vi "Butterfly_PullDown RC2_wCap_ERMod.vi"(0 "Semiconductor Module Context":T2, 1 "RFPins":string[](array[string]), 2 "current level":dbl=0.01 format="%_6p", 3 "R Thresholds":dbl[](array[numeric]), 5 "error in (no error)":errorcluster, 6 "PD_Pin":string="SMU_PD", 7 "Start_v":dbl=10.0 format="%#_13g", 9 "Stop_v":dbl=41.0 format="%#_13g", 10 "VNAs Measurement Parameters":T1, 11 "Step_v":dbl=1.0) -> (14 "Semiconductor Module Context Out":T2, 19 "error out":errorcluster)   [LabVIEW 2013]
uses:
  <vilib>/NI_TestStand_SemiconductorModule/NI_TestStand_Semiconductor_Module.lvlibp/PinMap/General/SemiconductorModuleContext.ctl
  VNA/VNAs Measurement Parameters.ctl
  <instrlib>/niDCPower/nidcpower.llb/niDCPower Wait For Event - Event.ctl
  <vilib>/NI_TestStand_SemiconductorModule/NI_TestStand_Semiconductor_Module.lvlibp/PinMap/DC Power/PinToNIDCPowerSession.vi
  <vilib>/NI_TestStand_SemiconductorModule/NI_TestStand_Semiconductor_Module.lvlibp/PinMap/DC Power/PinsToNIDCPowerSessions.vi
  <vilib>/NI_TestStand_SemiconductorModule/NI_TestStand_Semiconductor_Module.lvlibp/PinMap/General/Publish/PublishDataDoubleFunctionalTest.vi
  <vilib>/NI_TestStand_SemiconductorModule/NI_TestStand_Semiconductor_Module.lvlibp
panel:
  out "Multisite Cap Data":dbl[][](array[numeric])
  out "Full R Array":dbl[][][](array[numeric])
  out "step":i32
  out "Instrument Session":refnum<k15>
  out "sites and pins loop iter":i32
  out "Channel List":string
  out "BF values":dbl[](array[numeric])
  out "BF Names":string[](array[string])
  out "R Array":dbl[](array[numeric])
  out "BFSamples":i32
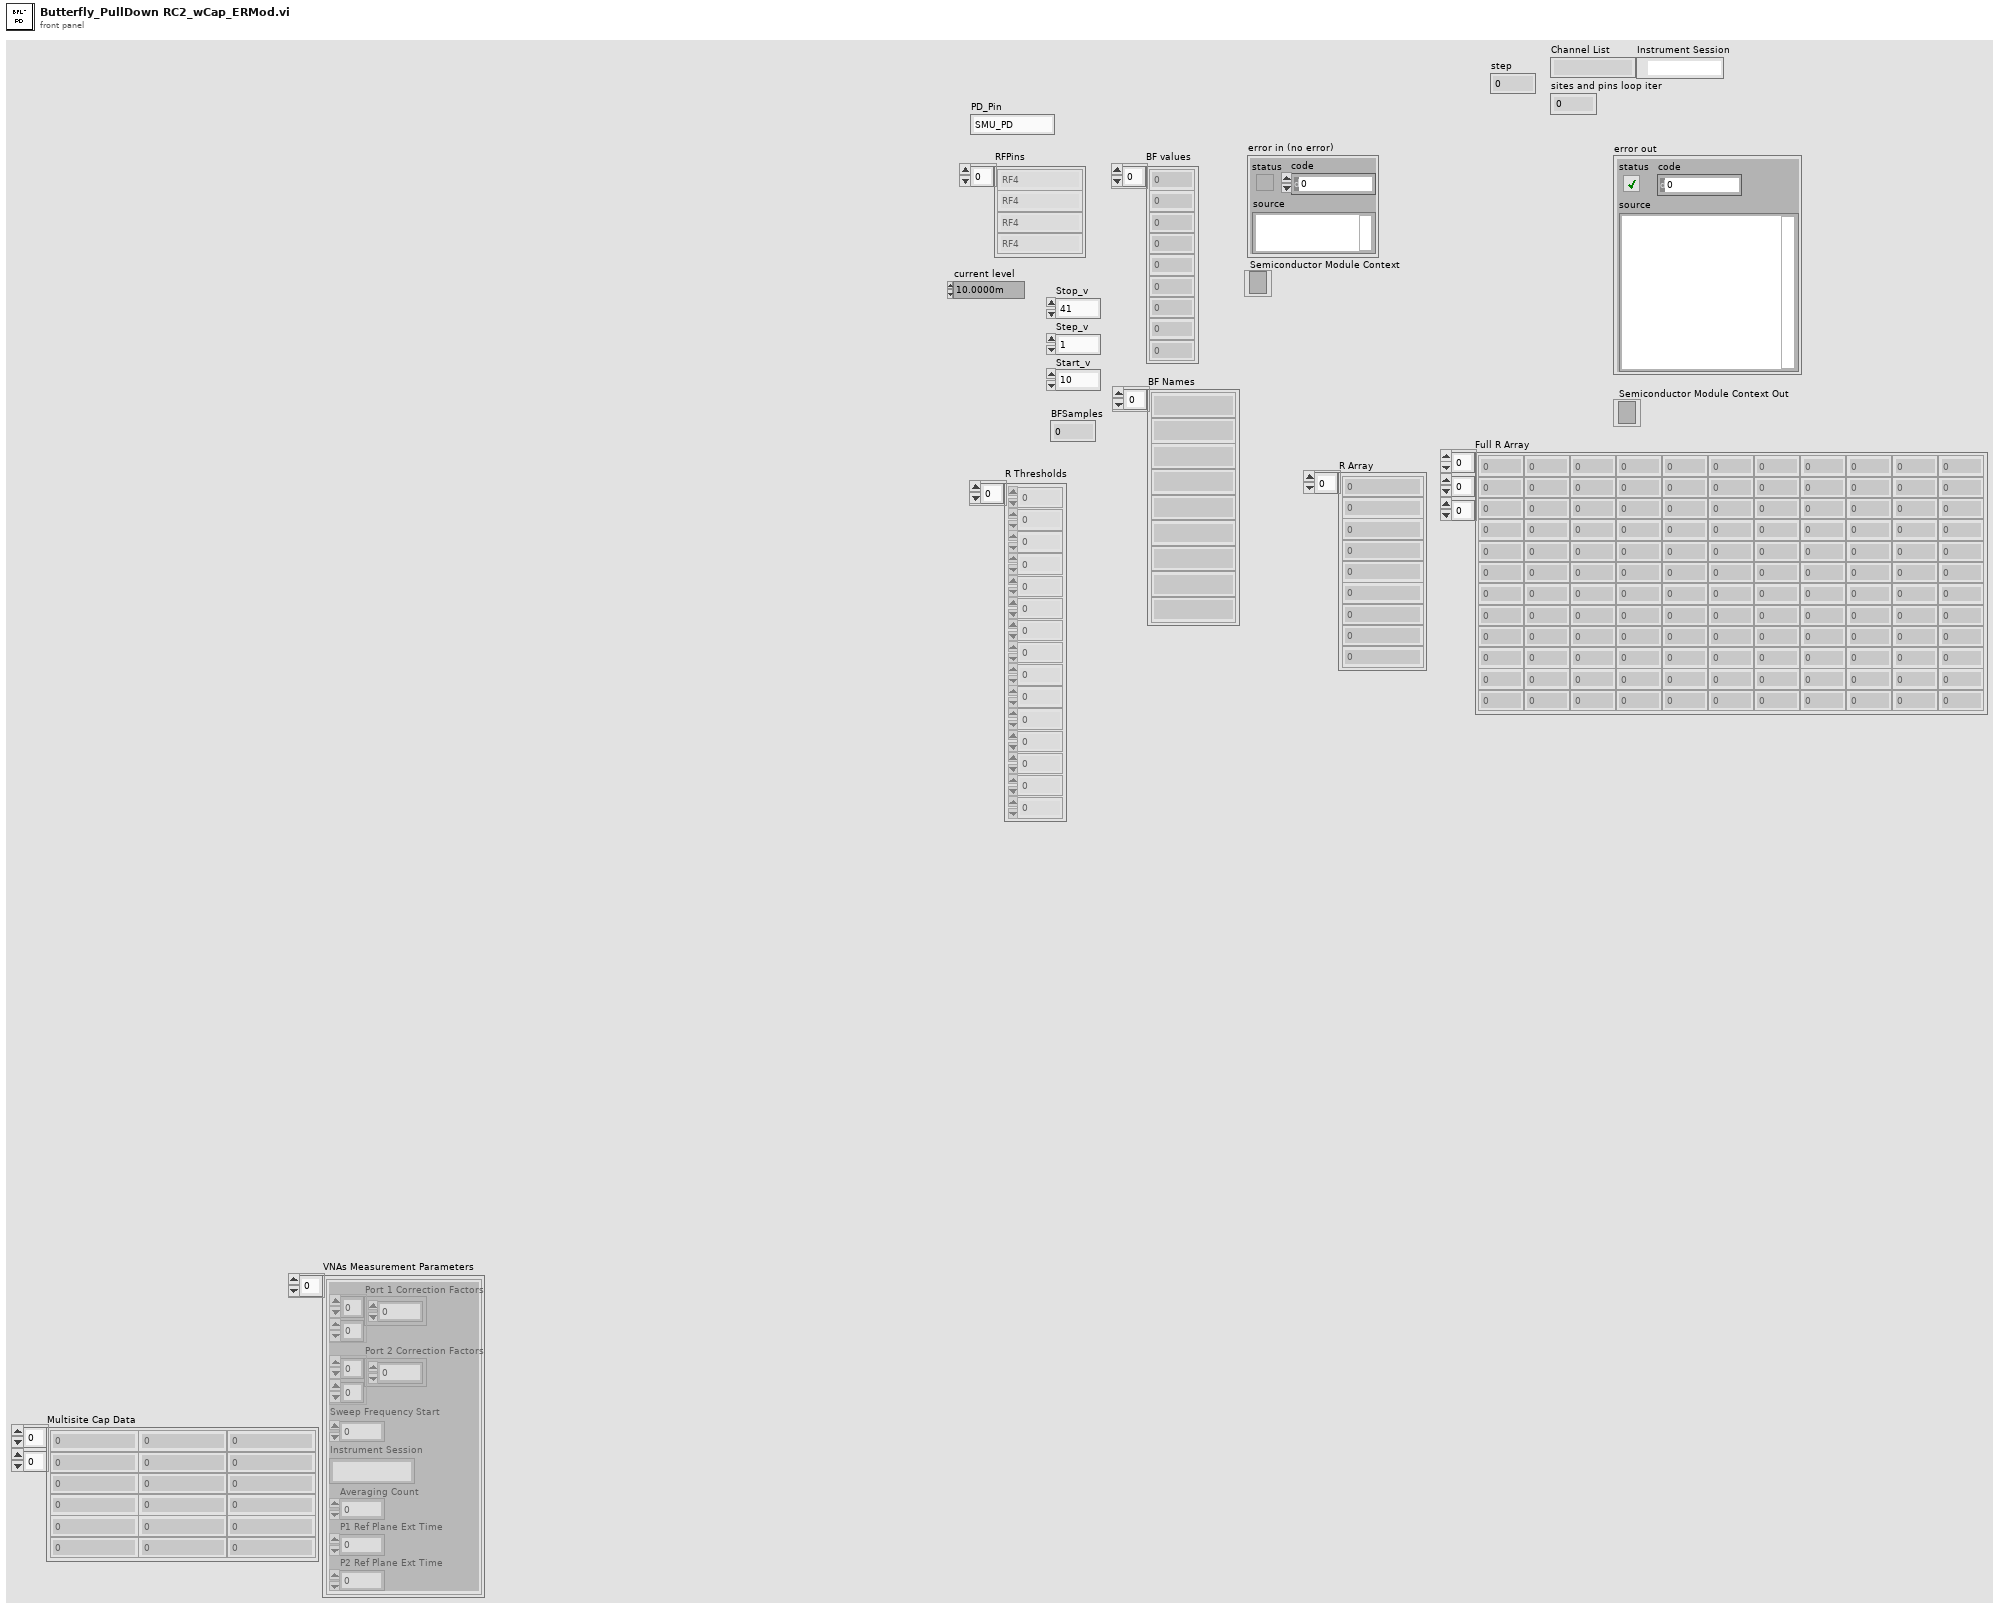
[diagram p1: front panel]
types:
  T1 = typedef "VNAs Measurement Parameters.ctl" = cluster{"Port 1 Correction Factors":cdb[][], "Port 2 Correction Factors":cdb[][], "Sweep Frequency Start":dbl, "Instrument Session":string, "Averaging Count":i32, "P1 Ref Plane Ext Time":dbl, "P2 Ref Plane Ext Time":dbl}[]
  T2 = typedef "NI_TestStand_Semiconductor_Module.lvlibp/SemiconductorModuleContext.ctl" = refnum<k7>
  T3 = typedef "niDCPower Wait For Event - Event.ctl" = i32
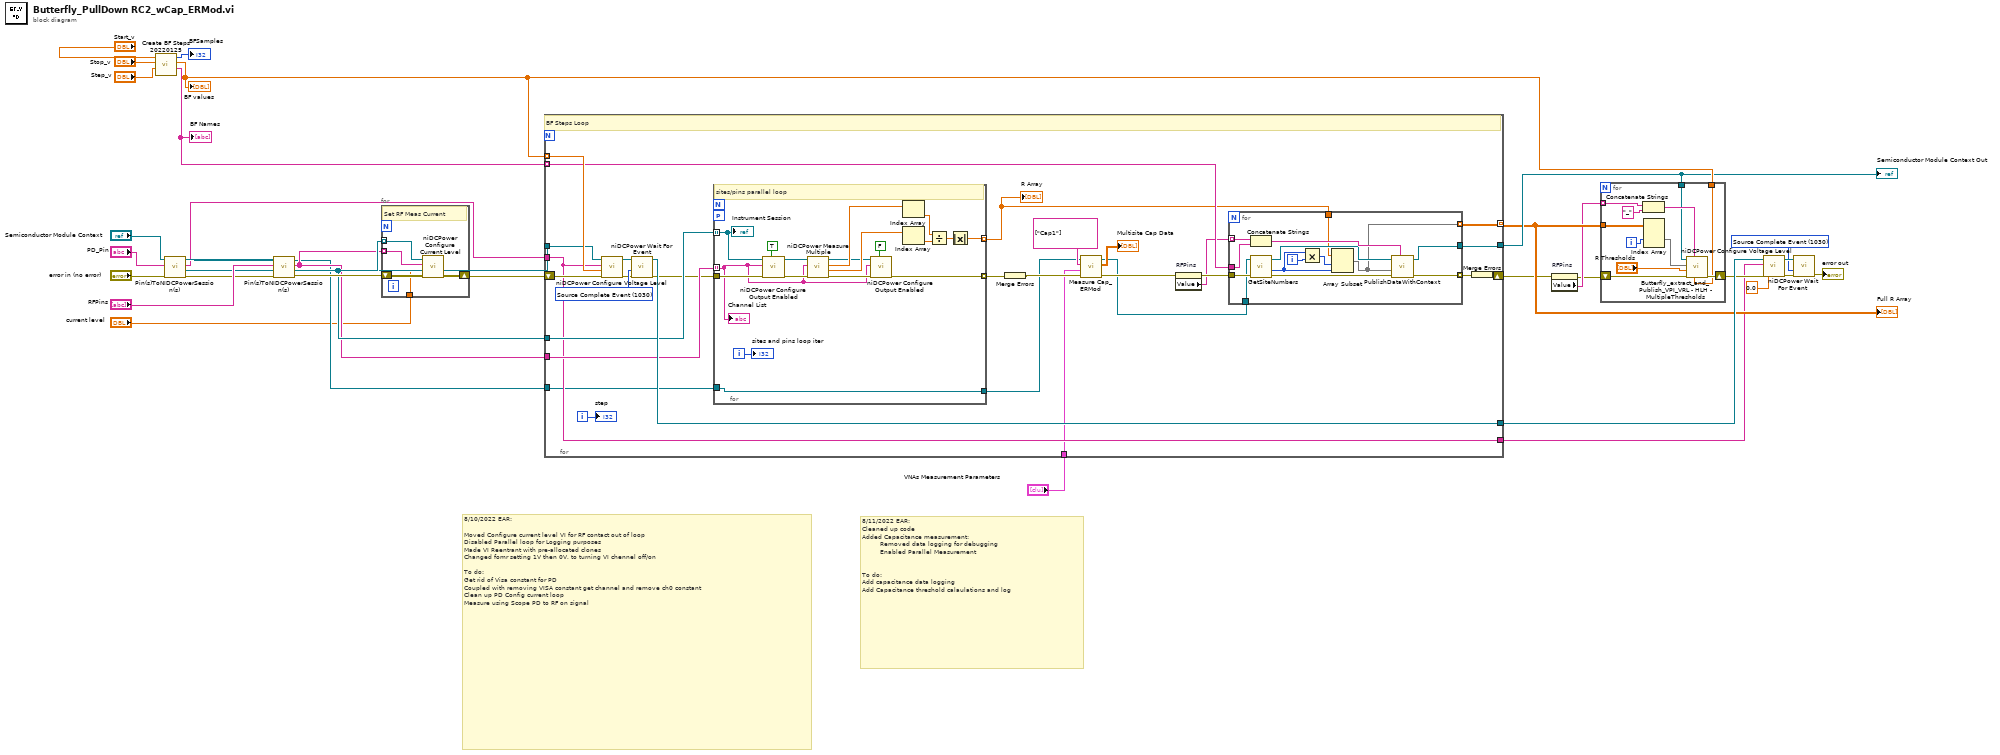
[diagram p0: block diagram]
diagram:
  w25 = T3 1030 items=["Source Complete Event"=1030, "Measure Complete Event"=1031, "Sequence Iteration Complete Event"=1032, "Sequence Engine Done Event"=1033, "Pulse Complete Event"=1051, "Ready For Pulse Trigger Event"=1052] ("event")
  # "8/11/2022 EAR:\nCleaned up code\nAdded Capacitance measurement:\n         Removed data logging for debugging\n         Enabled Parallel Measurement\n\n\nTo do:\nAdd capacitance data logging\nAdd Capacitance threshold calaulations and log"
  # "8/10/2022 EAR:\n\nMoved Configure current level VI for RF contact out of loop\nDisabled Parallel loop for Logging purposes\nMade VI Reentrant with pre-allocated clones\nChanged fomr setting 1V then 0V, to turning VI chennel off/on\n\nTo do:\nGet rid of Visa constant for PD\nCoupled with removing VISA constant get channel and remove ch0 constant\nClean up PD Config current loop\nMeasure using Scope PD to RF on signal"
  n1 = call "Create BF Steps 20220125.vi"("Step_v"="Step_v", "Stop_v"="Stop_v", "Start_v"="Start_v") -> ("BF Names"=w24:string[], "BF values"=w23:dbl[], "BFSamples"=→"BFSamples":i32)  [unwired: 6 in]
  "BF Names" <- w24
  "BF values" <- w23
  n2 = call-poly <vilib>:"Pin(s)ToNIDCPowerSession(s).vi"("error in (no error)"="error in (no error)", "Pin"="PD_Pin", "Semiconductor Module Context"="Semiconductor Module Context") -> ("error out"=w11:errorcluster, "Instrument Session"=w8:refnum<k15>, "Channel List"=w7:string, "Semiconductor Module Context Out"=w12:T2)  [unwired: 4 in, 1 out]
  n3 = call-poly <vilib>:"Pin(s)ToNIDCPowerSession(s).vi"("error in (no error)"=w11, "Pins"="RFPins", "Semiconductor Module Context"=w12) -> ("error out"=w20:errorcluster, "Instrument Sessions"=w18:refnum<k15>[], "Channel Lists"=w17:string[], "Semiconductor Module Context Out"=w15:T2)  [unwired: 4 in, 1 out]
  n4 = for {
    shift-right: [w38] -> w19
    shift-left: w20 -> [w39]
    tunnel: w18 -> [w37] mode=indexing
    tunnel: w17 -> [w36] mode=indexing
    tunnel: "current level" -> [w35]
    # "Set RF Meas Current"
    n5 = call <instrlib>:"niDCPower Configure Current Level.vi"("error in (no error)"=w39, "current level"=w35, "channel name"=w36, "instrument handle"=w37) -> ("error out"=w38:errorcluster)  [unwired: 6 in, 1 out]
  }
  n6 = for {
    shift-right: [w57] -> w4
    shift-left: w19 -> [w65]
    tunnel: w23 -> [w64] mode=indexing
    tunnel: w8 -> [w63]
    tunnel: [w62] -> w29
    tunnel: w24 -> [w59] mode=indexing
    tunnel: [w58] -> w21
    tunnel: w18 -> [w56]
    tunnel: w17 -> [w55]
    tunnel: w15 -> [w47]
    tunnel: [w52] -> w14 mode=indexing
    tunnel: w7 -> [w48]
    tunnel: [w48] -> w2
    tunnel: "VNAs Measurement Parameters" -> [w40]
    i -> [w61]
    w67 = T3 1030 items=["Source Complete Event"=1030, "Measure Complete Event"=1031, "Sequence Iteration Complete Event"=1032, "Sequence Engine Done Event"=1033, "Pulse Complete Event"=1051, "Ready For Pulse Trigger Event"=1052] ("event")
    # "BF Steps Loop"
    n7 = call <instrlib>:"niDCPower Configure Voltage Level.vi"("error in (no error)"=w65, "voltage level"=w64, "channel name"=w48, "instrument handle"=w63) -> ("error out"=w66:errorcluster, "instrument handle out"=w68:refnum<k15>)  [unwired: 6 in]
    n8 = call <instrlib>:"niDCPower Wait For Event.vi"("error in (no error)"=w66, "event"=w67, "instrument handle"=w68) -> ("error out"=w54:errorcluster, "instrument handle out"=w62:refnum<k15>)  [unwired: 7 in]
    n9 = for {
      workers-P: _ -> [_]
      tunnel: w56 -> [w90] mode=indexing
      tunnel: w55 -> [w86] mode=indexing
      tunnel: [w85] -> w53 mode=indexing
      tunnel: w54 -> [w94]
      tunnel: [w84] -> w51 mode=indexing
      tunnel: w47 -> [w83]
      tunnel: [w83] -> w42
      i -> [w100]
      # "sites/pins parallel loop"
      n10 = call <instrlib>:"niDCPower Configure Output Enabled.vi"("error in (no error)"=w94, "output enabled"=TRUE, "channel name"=w86, "instrument handle"=w90) -> ("error out"=w92:errorcluster, "instrument handle out"=w91:refnum<k15>)  [unwired: 6 in]
      n11 = call <instrlib>:"niDCPower Measure Multiple.vi"("error in (no error)"=w92, "channel name"=w86, "instrument handle"=w91) -> ("error out"=w89:errorcluster, "current measurements"=w99:dbl[], "voltage measurements"=w98:dbl[], "instrument handle out"=w87:refnum<k15>)  [unwired: 5 in]
      n12 = call <instrlib>:"niDCPower Configure Output Enabled.vi"("error in (no error)"=w89, "output enabled"=FALSE, "channel name"=w86, "instrument handle"=w87) -> ("error out"=w84:errorcluster)  [unwired: 6 in, 1 out]
      n13 = Index Array(array=w98) -> (element=w96:dbl)  [unwired: 1 in]
      n14 = Index Array(array=w99) -> (element=w97:dbl)  [unwired: 1 in]
      n15 = Divide(x=w96, y=w97) -> (x/y=w95:dbl)
      n16 = Absolute Value(x=w95) -> (abs(x)=w85:dbl)
      "Channel List" <- w86
      "sites and pins loop iter" <- w100
      "Instrument Session" <- w90
    }
    "R Array" <- w53
    n17 = Merge Errors(w51) -> (w44:errorcluster)
    n18 = call "Measure Cap_ERMod.vi"("error in (no error)"=w44, "VNAs Measurement Parameters"=w40, "Pins"=string[] ["Cap1"] ("Capacitance Pins"), "Semiconductor Module Context"=w42) -> ("error out"=w43:errorcluster, "Multisite Cap Data"=→"Multisite Cap Data":dbl[][], "Semiconductor Module Context Out"=w41:T2)  [unwired: 5 in]
    n19 = property on="RFPins" class="Arr (strict)"(error in=w43) -> (error out=w50:errorcluster, "Value"=w49:string[])  [unwired: 1 in, 1 out]
    n20 = for {
      tunnel: [w78] -> w60 mode=indexing
      tunnel: w49 -> [w81] mode=indexing
      tunnel: w59 -> [w80]
      tunnel: w50 -> [w72]
      tunnel: [w76] -> w58
      tunnel: w53 -> [w71]
      tunnel: w41 -> [w70]
      tunnel: [w69] -> w52 mode=indexing
      i -> [w82]
      n21 = Concatenate Strings(w81, w80) -> (w77:string)
      n22 = call <vilib>:"GetSiteNumbers.vi"("error in (no error)"=w72, "Semiconductor Module Context"=w70) -> ("error out"=w75:errorcluster, "Number Of Sites"=w73:i32, "Semiconductor Module Context Out"=w74:T2)  [unwired: 6 in, 1 out]
      n23 = Multiply(x=w73, y=w82) -> (x*y=w79:i32)
      n24 = Array Subset(array=w71, index=w79, length=w73) -> (w69:dbl[])
      n25 = call-poly <vilib>:"PublishDataWithContext.vi"("Published Data Id"=w77, "error in (no error)"=w75, "Data In"=w69, "Semiconductor Module Context"=w74) -> ("error out"=w78:errorcluster, "Semiconductor Module Context Out"=w76:T2)  [unwired: 6 in]
    }
    n26 = Merge Errors(w60) -> (w57:errorcluster)
    "step" <- w61
  }
  "Semiconductor Module Context Out" <- w21
  "Full R Array" <- w14
  n27 = property on="RFPins" class="Arr (strict)"(error in=w4) -> (error out=w3:errorcluster, "Value"=w5:string[])  [unwired: 1 in, 1 out]
  n28 = for {
    tunnel: w5 -> [w107] mode=indexing
    shift-right: [w108] -> w22
    shift-left: w3 -> [w109]
    tunnel: w21 -> [w104]
    tunnel: w23 -> [w103]
    tunnel: w14 -> [w102]
    i -> [w111]
    n29 = Concatenate Strings(w107, "_" ("string")) -> (w105:string)
    n30 = Index Array(array=w102, index (dim 1)=w111) -> (element=w101:dbl[][])  [unwired: 2 in]
    n31 = call "Butterfly_extract_and_Publish_VPI_VRL - HLH - MultipleThresholds.vi"("Voltages Array"=w103, "ID Prefix"=w105, "error in (no error)"=w109, "Thresholds"="R Thresholds", "Result Array In"=w101, "Semiconductor Module Context"=w104) -> ("error out"=w108:errorcluster)  [unwired: 5 in]
  }
  n32 = call <instrlib>:"niDCPower Configure Voltage Level.vi"("error in (no error)"=w22, "voltage level"=0.0, "channel name"=w2, "instrument handle"=w29) -> ("error out"=w28:errorcluster, "instrument handle out"=w26:refnum<k15>)  [unwired: 6 in]
  n33 = call <instrlib>:"niDCPower Wait For Event.vi"("error in (no error)"=w28, "event"=w25, "instrument handle"=w26) -> ("error out"=→"error out":errorcluster)  [unwired: 7 in, 1 out]
